vi "Create TestComplete Reader.vi"(6 "Station":T1(ring), 8 "error in (no error)":errorcluster) -> (0 "error out":errorcluster, 3 "reader endpoint":refnum<k21>)   [LabVIEW 2019, in "Test Bench Tools.lvlib"]
uses:
  Test Bench Tools.lvlib
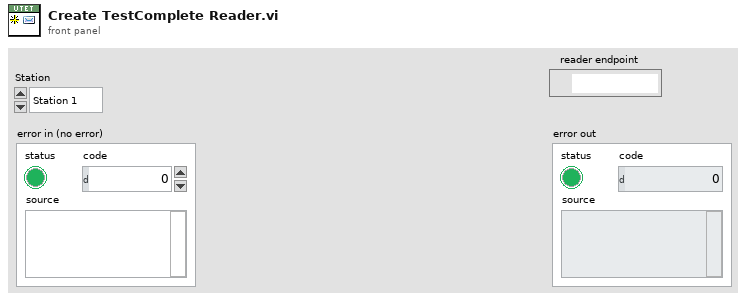
[diagram p1: front panel]
types:
  T1 = enum16{"Station 1", "Station 2", "Station 3", "Station 4"}
  T2 = cluster{"Socket":i32, "SerialNumber":string, "TestResult":string}
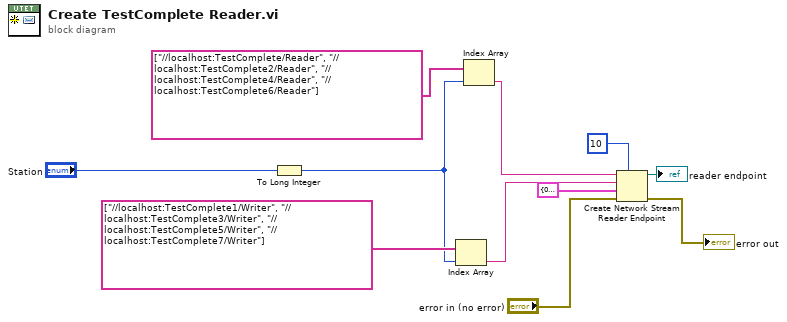
[diagram p0: block diagram]
diagram:
  n1 = To Long Integer(number="Station") -> (32bit integer=w2:i32)
  n2 = Index Array(array=string[] ["//localhost:TestComplete1/Writer", "//localhost:TestComplete3/Writer", "//localhost:TestComplete5/Writer", "//localhost:TestComplete7/Writer"], index=w2) -> (element=w1:string)
  n3 = Index Array(array=string[] ["//localhost:TestComplete/Reader", "//localhost:TestComplete2/Reader", "//localhost:TestComplete4/Reader", "//localhost:TestComplete6/Reader"], index=w2) -> (element=w5:string)
  n4 = Create Network Stream Reader Endpoint(7:10 ("reader buffer size"), 8:"error in (no error)", 9:T2 {"Socket"=0, "SerialNumber"="", "TestResult"=""}, 10:w1, 11:w5) -> (0:→"error out":errorcluster, 3:→"reader endpoint":refnum<k21>)  [unwired: 2 in]
